vi "EX1.vi"() -> ()   [LabVIEW 2018]
panel:
  out "A+B":dbl
  in  "B":dbl
  in  "A":dbl
  out "date string":string
  out "time string":string
  # "EX1 - TP0"
  # "Mekni Marwen 2ème Année Génie Electrique"
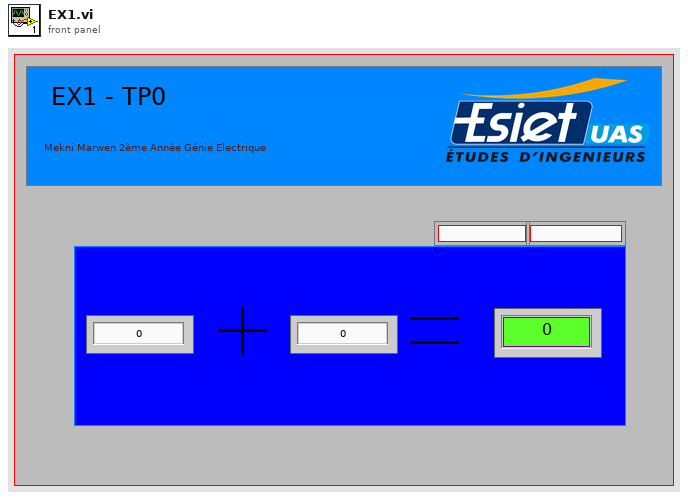
[diagram p1: front panel]
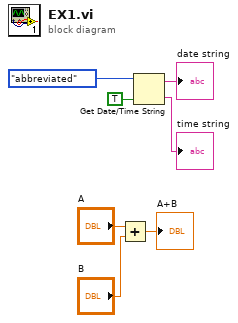
[diagram p0: block diagram]
diagram:
  n1 = Add(x="A", y="B") -> (x+y=→"A+B":dbl)
  n2 = Get Date/Time String(date format (0)=enum16{"short", "long", "abbreviated"}."abbreviated", want seconds? (F)=TRUE) -> (date string=→"date string":string, time string=→"time string":string)  [unwired: 1 in]
